vi "Initialize.vi"   [LabVIEW 2014, in "Hokuyo URG Series.lvlib"]
uses:
  Hokuyo URG Series.lvlib
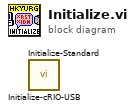
[diagram p0: block diagram]
diagram:
  n1 = call "Initialize-cRIO-USB.vi"() -> ()  [unwired: 10 in, 2 out]
  n2 = call "Initialize-Standard.vi"() -> ()  [unwired: 10 in, 2 out]
